vi "Main.vi"(8 "error in (no error)":errorcluster) -> (0 "error out":errorcluster)   [LabVIEW 2022 SP3, in "VMR-Deck.lvlib" / "App.lvclass"]
uses:
  App.lvclass
  App.lvclass/App.ctl
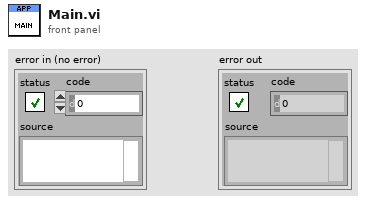
[diagram p1: front panel]
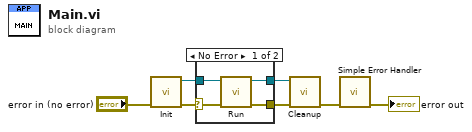
[diagram p0: block diagram]
diagram:
  n1 = call "Init.vi"("error in (no error)"="error in (no error)") -> ("error out"=w6:errorcluster, "App out"=w5:refnum<class "App.lvclass">)  [unwired: 9 in]
  n2 = case shown="No Error" w6 {
    selector: w6 -> [w10 w12]
    tunnel: w5 -> [w11 w13]
    tunnel: [w8 w13] -> w3
    tunnel: [w9 w12] -> w4
    frame No Error {
      n3 = call "Run.vi"("error in (no error)"=w10, "App in"=w11) -> ("error out"=w9:errorcluster, "App out"=w8:refnum<class "App.lvclass">)  [unwired: 8 in]
    }
    frame Error {
    }
  }
  n4 = call "Cleanup.vi"("error in (no error)"=w4, "App in"=w3) -> ("error out"=w2:errorcluster)  [unwired: 9 in]
  n5 = call <vilib>:"Simple Error Handler.vi"("error in (no error)"=w2) -> ("error out"=→"error out":errorcluster)  [unwired: 4 in, 4 out]
